vi "START5PYTHONEHHHHHH.vi"() -> ()   [LabVIEW 2024]
uses:
  <vilib>/Utility/file.llb/Read Delimited Spreadsheet (DBL).vi
panel:
  in  "Desired Flow Rate":dbl
  in  "Initial RPM Value":dbl
  out "Right Heart Waveform":dbl[](graph)
  out "LVAD Speed Waveform":dbl[](graph)
  out "Flow Rate Waveform":dbl[](graph)
  in  "stop":bool
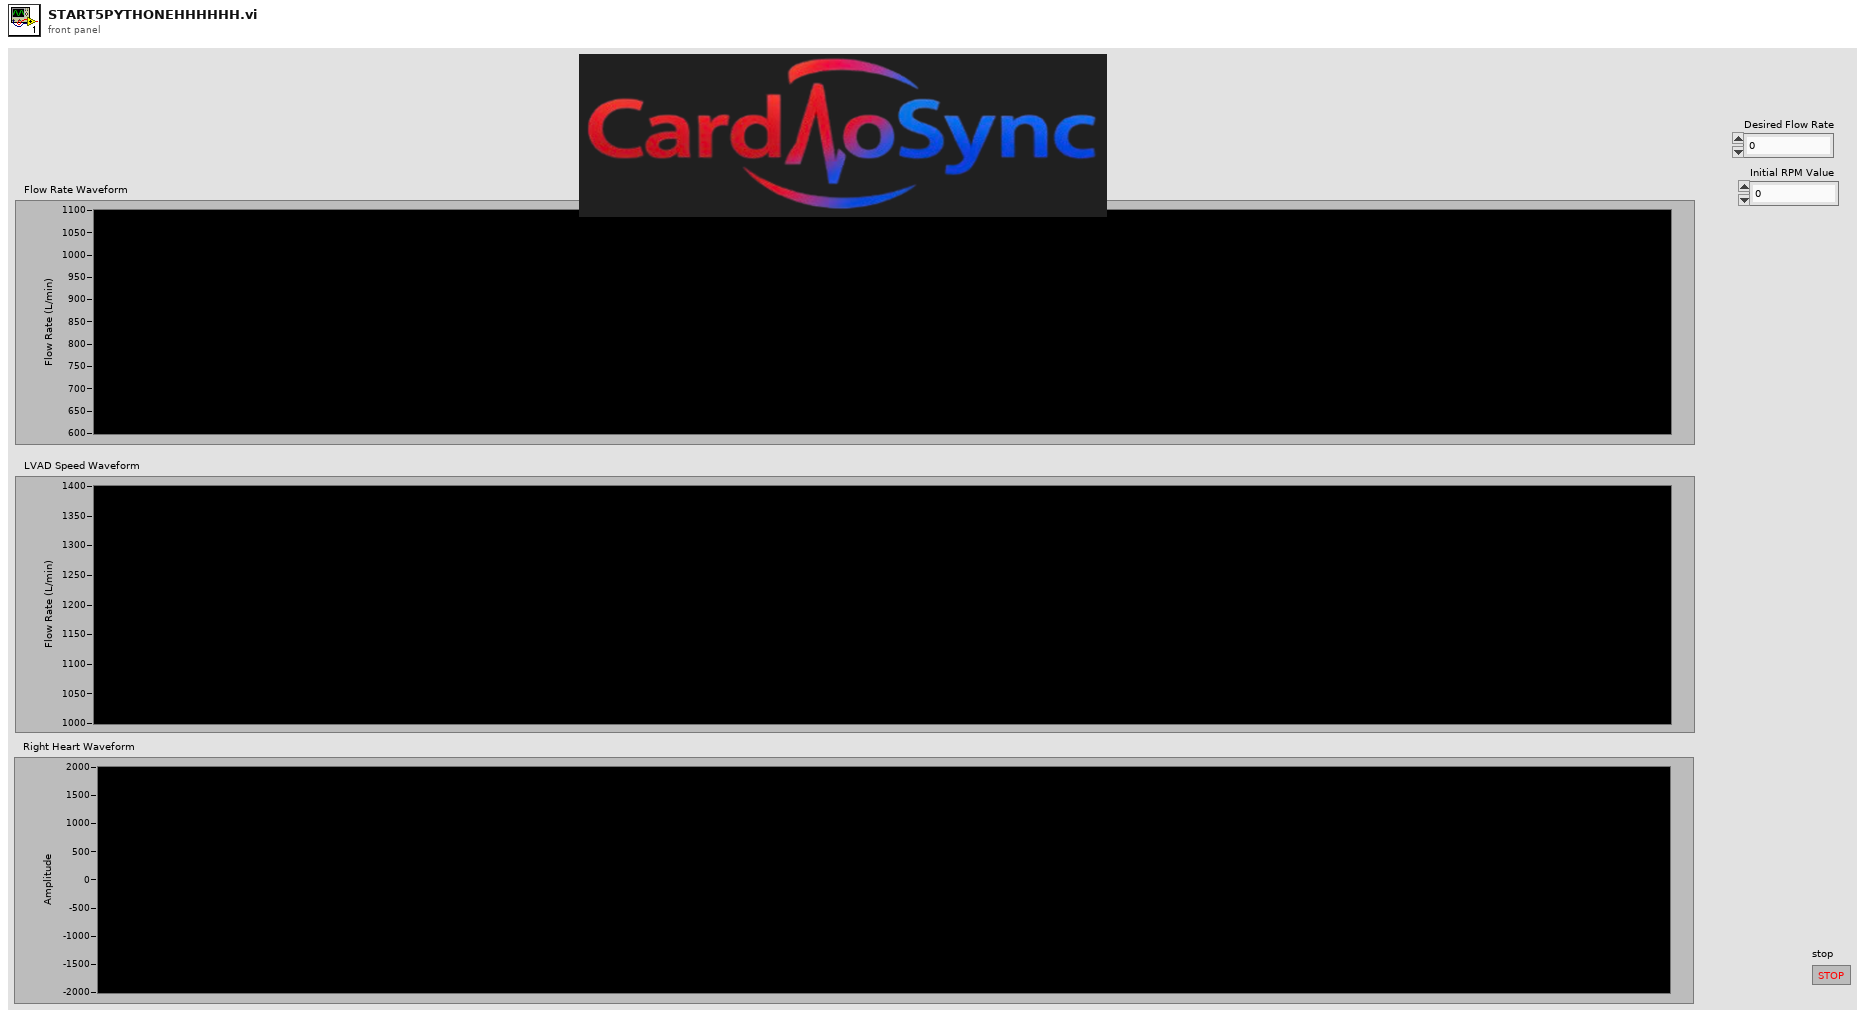
[diagram p1: front panel]
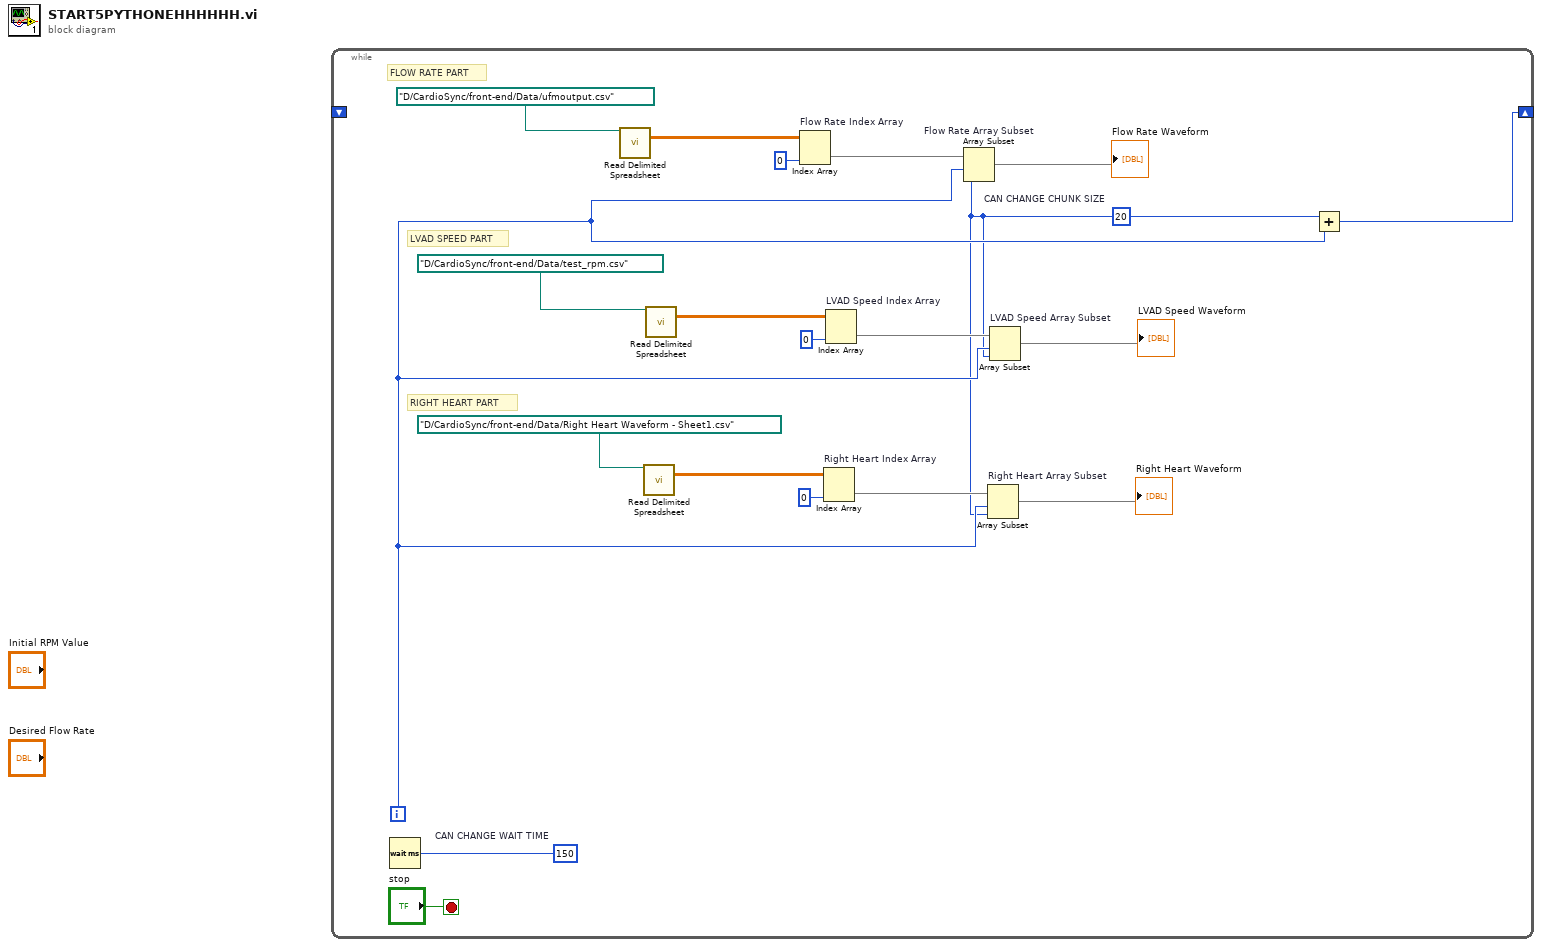
[diagram p0: block diagram]
diagram:
  n1 = while {
    shift-right: [w15] -> _
    shift-left: _ -> [_]
    i -> [w3]
    stop <- "stop" stop-if-true
    w16 = u32 150  # CAN CHANGE WAIT TIME
    w2 = 20  # CAN CHANGE CHUNK SIZE
    # "RIGHT HEART PART"
    # "LVAD SPEED PART"
    # "FLOW RATE PART"
    n2 = Wait (ms)(milliseconds to wait=w16) -> ()  [unwired: 1 out]
    n3 = call-poly <vilib>:"Read Delimited Spreadsheet.vi"("file path (dialog if empty)"=path "D:/CardioSync/front-end/Data/ufmoutput.csv") -> ("all rows"=w18:dbl[][])  [unwired: 9 in, 5 out]
    n4 = call-poly <vilib>:"Read Delimited Spreadsheet.vi"("file path (dialog if empty)"=path "D:/CardioSync/front-end/Data/Right Heart Waveform - Sheet1.csv") -> ("all rows"=w6:dbl[][])  [unwired: 9 in, 5 out]
    n5 = call-poly <vilib>:"Read Delimited Spreadsheet.vi"("file path (dialog if empty)"=path "D:/CardioSync/front-end/Data/test_rpm.csv") -> ("all rows"=w10:dbl[][])  [unwired: 9 in, 5 out]
    n6 = Index Array "Flow Rate Index Array"(array=w18, index (col)=0 ("disabled index (col)")) -> (element=w17:dbl[])  [unwired: 1 in]
    n7 = Index Array "Right Heart Index Array"(array=w6, index (col)=0 ("disabled index (col)")) -> (element=w5:dbl[])  [unwired: 1 in]
    n8 = Index Array "LVAD Speed Index Array"(array=w10, index (col)=0 ("disabled index (col)")) -> (element=w9:dbl[])  [unwired: 1 in]
    n9 = Array Subset "Flow Rate Array Subset"(array=w17, index=w3, length=w2) -> (→"Flow Rate Waveform":dbl[])
    n10 = Array Subset "Right Heart Array Subset"(array=w5, index=w3, length=w2) -> (→"Right Heart Waveform":dbl[])
    n11 = Array Subset "LVAD Speed Array Subset"(array=w9, index=w3, length=w2) -> (→"LVAD Speed Waveform":dbl[])
    n12 = Add(x=w2, y=w3) -> (x+y=w15:i32)
  }
